vi "event.create.vi"(7 "Time Stamp (now)":timestamp format="%<%x %.3X>T", 8 "error in":errorcluster, 9 "Type":enum16{"INFO", "FLAG", "ERROR", "SUCCESS"}(ring), 10 "Name":string, 11 "asset in":refnum<class "asset.lvclass">) -> (0 "error out":errorcluster, 2 "event":refnum<class "event.lvclass">, 3 "asset out":refnum<class "asset.lvclass">)   [LabVIEW 2020, in "asset.lvclass"]
uses:
  asset.lvclass
  event/event.lvclass
  asset.lvclass/asset.ctl
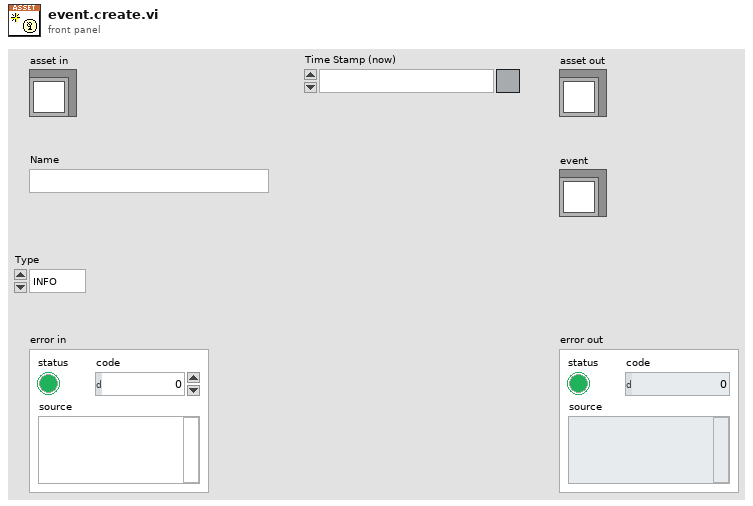
[diagram p1: front panel]
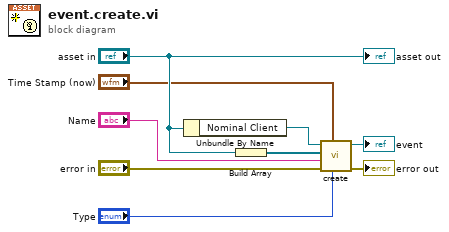
[diagram p0: block diagram]
diagram:
  n1 = Unbundle By Name("asset in") -> ("Nominal Client"=w9:refnum<class "Nominal Client.lvclass">)
  n2 = Build Array("asset in") -> (w8:refnum<class "asset.lvclass">[])
  n3 = call "create.vi"("Type"="Type", "Time Stamp (now)"="Time Stamp (now)", "error in"="error in", "Name"="Name", "assets"=w8, "Nominal Client in"=w9) -> ("error out"=→"error out":errorcluster, "event"=→"event":refnum<class "event.lvclass">)  [unwired: 4 in]
  "asset out" <- "asset in"
